vi "LEUI.vi"(0 "LED Update Rate (s)":dbl=0.25 caption="Delay Time (s)", 6 "LEUI_Buttons":T1={"Cycle Selection"=enum."Cycle 0", "SW302 - Option"=TRUE, "SW301 - Start/Pause"=FALSE, "Cycle Selection"=enum."Cycle 0", "Number of positions 1"=2, "Knob Position 1"=0, "Number of positions 2"=2, "Knob Position 2"=0, "Number of positions 3"=2, "Knob Position 3"=0, "Number of positions 4"=2, "Knob Position 4"=0} {"Knob Position 4" items=["Six"=5, "Five"=4, "Four"=3, "Three"=2, "Two"=1, "One"=0]; "Number of positions 4" items=["Six"=5, "Five"=4, "Four"=3, "Three"=2]; "Knob Position 3" items=["Six"=5, "Five"=4, "Four"=3, "Three"=2, "Two"=1, "One"=0]; "Number of positions 3" items=["Six"=5, "Five"=4, "Four"=3, "Three"=2]; "Knob Position 2" items=["Six"=5, "Five"=4, "Four"=3, "Three"=2, "Two"=1, "One"=0]; "Number of positions 2" items=["Six"=5, "Five"=4, "Four"=3, "Three"=2]; "Knob Position 1" items=["Six"=5, "Five"=4, "Four"=3, "Three"=2, "Two"=1, "One"=0]; "Number of positions 1" items=["Six"=5, "Five"=4, "Four"=3, "Three"=2]}, 7 "stop":bool, 11 "Error In":errorcluster) -> (15 "Error Out":errorcluster)   [LabVIEW 2014]
doc: "This VI controls the high end 2015 VA washer UI board. The VI updates the status of the LEDs every 'LED update rate (s)' number of seconds. The VI allows the user to press buttons and select a cycle."
uses:
  Laundry Tool 1.0 Support/type defs/LEUI_Buttons.ctl
  Laundry Tool 1.0 Support/type defs/LEUI_LEDs_SLB.ctl
  Common/LabVIEW GEA2 Toolkit/LabVIEW_GEA2_Toolkit.lvlibp/type defs/Data In.ctl
  Common/LabVIEW GEA2 Toolkit/LabVIEW_GEA2_Toolkit.lvlibp/type defs/Source_Destination.ctl
  Common/LabVIEW GEA2 Toolkit/LabVIEW_GEA2_Toolkit.lvlibp/type defs/ERD Read Data In.ctl
  Common/LabVIEW GEA2 Toolkit/LabVIEW_GEA2_Toolkit.lvlibp/type defs/Data Type.ctl
  Common/LabVIEW GEA2 Toolkit/LabVIEW_GEA2_Toolkit.lvlibp/type defs/ERD Write Data In.ctl
  Automation/Product Specific/Clothes Care/2015 VA Washer/Product Testcode/VALEW/Valew Common/type defs/UI Buttons.ctl
  Automation/Product Specific/Clothes Care/2015 VA Washer/Product Testcode/VALEW/Valew Common/type defs/Encoder Position.ctl
  Common/LabVIEW GEA2 Toolkit/LabVIEW_GEA2_Toolkit.lvlibp
panel:
  in  "Soft Load box?":bool
  out "LEUI_LEDs_Out":T2
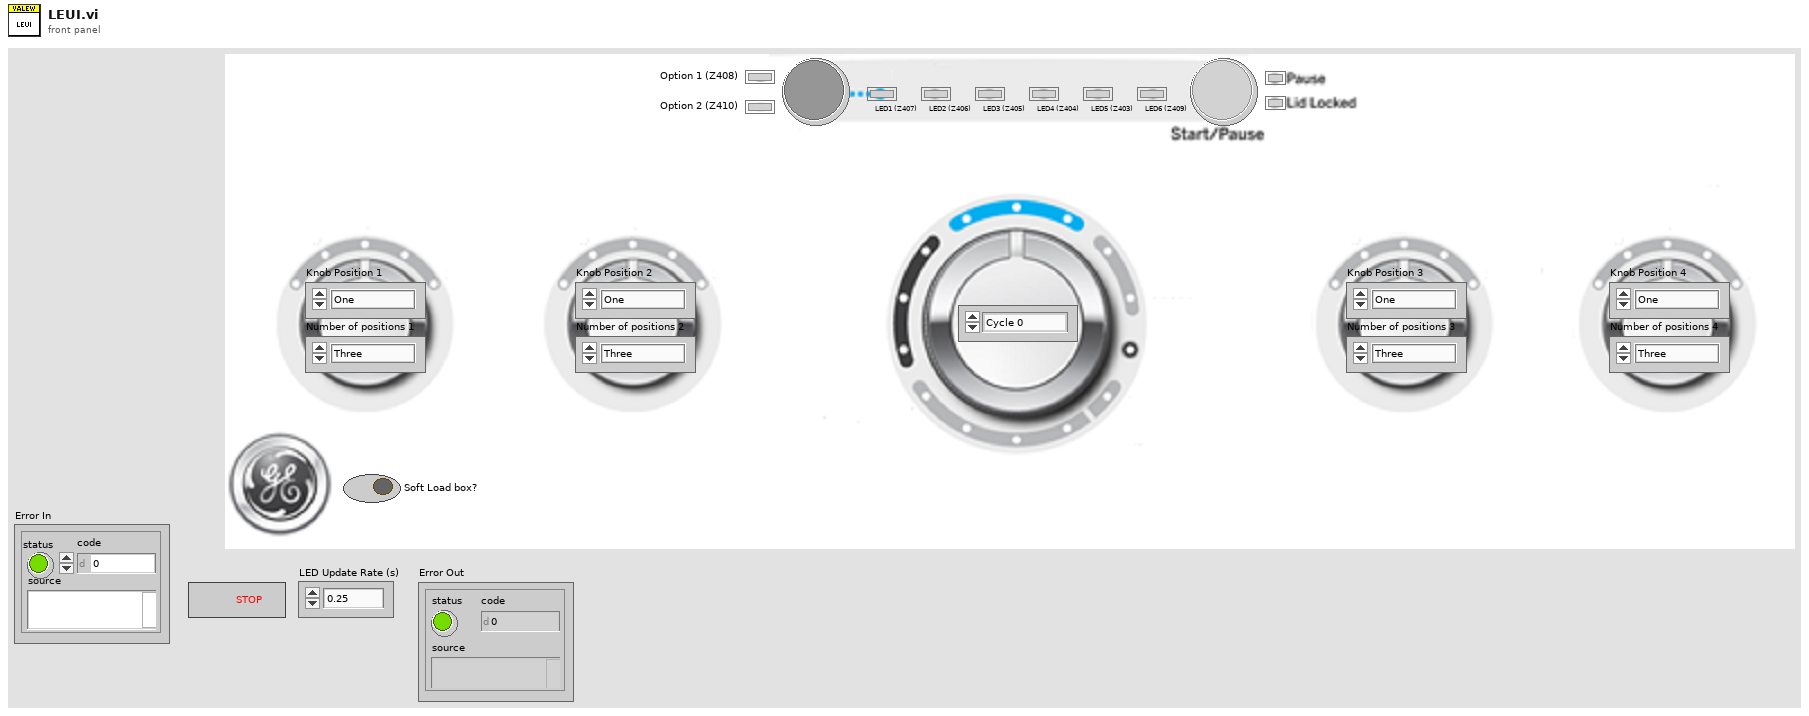
[diagram p1: front panel]
types:
  T1 = typedef "LEUI_Buttons.ctl" = cluster{"Cycle Selection":enum16{"Cycle 0", "Cycle 1", "Cycle 2", "Cycle 3", "Cycle 4", "Cycle 5", "Cycle 6", "Cycle 7", "Cycle 8", "Cycle 9", "Cycle 10", "Cycle 11", "Cycle 12", "Cycle 13"}, "SW302 - Option":bool, "SW301 - Start/Pause":bool, "Cycle Selection":enum16{"Cycle 13", "Cycle 12", "Cycle 11", "Cycle 10", "Cycle 9", "Cycle 8", "Cycle 7", "Cycle 6", "Cycle 5", "Cycle 4", "Cycle 3", "Cycle 2", "Cycle 1", "Cycle 0"}, "Number of positions 1":i32, "Knob Position 1":i32, "Number of positions 2":i32, "Knob Position 2":i32, "Number of positions 3":i32, "Knob Position 3":i32, "Number of positions 4":i32, "Knob Position 4":i32}
  T2 = typedef "LEUI_LEDs_SLB.ctl" = cluster{"Pause (Z401)":bool, "Lid Locked (Z402)":bool, "LED1 (Z407)":bool, "LED2 (Z406)":bool, "LED3 (Z405)":bool, "LED4 (Z404)":bool, "LED5 (Z403)":bool, "LED6 (Z409)":bool, "Option 1 (Z408)":bool, "Option 2 (Z410)":bool}
  T3 = typedef "LabVIEW_GEA2_Toolkit.lvlibp/ERD Write Data In.ctl" = cluster{"ERD Number":u16, "Data Type":T4, "Data":string}
  T4 = typedef "LabVIEW_GEA2_Toolkit.lvlibp/Data Type.ctl" = enum16{"string", "boolean", "uint8_t", "uint16_t", "uint32_t", "uint64_t", "int8_t", "int16_t", "int32_t", "int64_t"}
  T5 = typedef "LabVIEW_GEA2_Toolkit.lvlibp/ERD Read Data In.ctl" = cluster{"ERD Number":u16, "Data Type":T4}
  T6 = typedef "LabVIEW_GEA2_Toolkit.lvlibp/Source_Destination.ctl" = cluster{"Source":u8, "Destination":u8}
  T7 = typedef "LabVIEW_GEA2_Toolkit.lvlibp/Data In.ctl" = cluster{"Source":u8, "Destination":u8, "Command":u8, "Message":string}
  T8 = typedef "UI Buttons.ctl" = enum16{"Switch Off", "SW201 - My Cycle", "SW202 - Delay Wash", "SW203 - Extra Rinse", "SW204 - Signal / Volume", "SW205 - Spin", "SW206 - Deep Rinse / Fab Soft", "SW207 - Soil", "SW208 - Auto Soak", "SW209 - Temp", "SW210 - Warm Rinse", "SW211 - Deep Fill", "SW212 - Stain Remover", "SW213 - Power", "SW222 - Control Lock", "SW214 - Start / Pause", "SW301 - Start/Pause LE", "SW302 - Option Button LE"}
  T9 = typedef "Encoder Position.ctl" = enum16{"Position 0", "Position 1", "Position 2", "Position 3", "Position 4", "Position 5", "Position 6", "Position 7", "Position 8", "Position 9", "Position 10", "Position 11", "Position 12", "Position 13", "Clear / Reset"}
  T10 = enum16{"Cycle 13", "Cycle 12", "Cycle 11", "Cycle 10", "Cycle 9", "Cycle 8", "Cycle 7", "Cycle 6", "Cycle 5", "Cycle 4", "Cycle 3", "Cycle 2", "Cycle 1", "Cycle 0"}
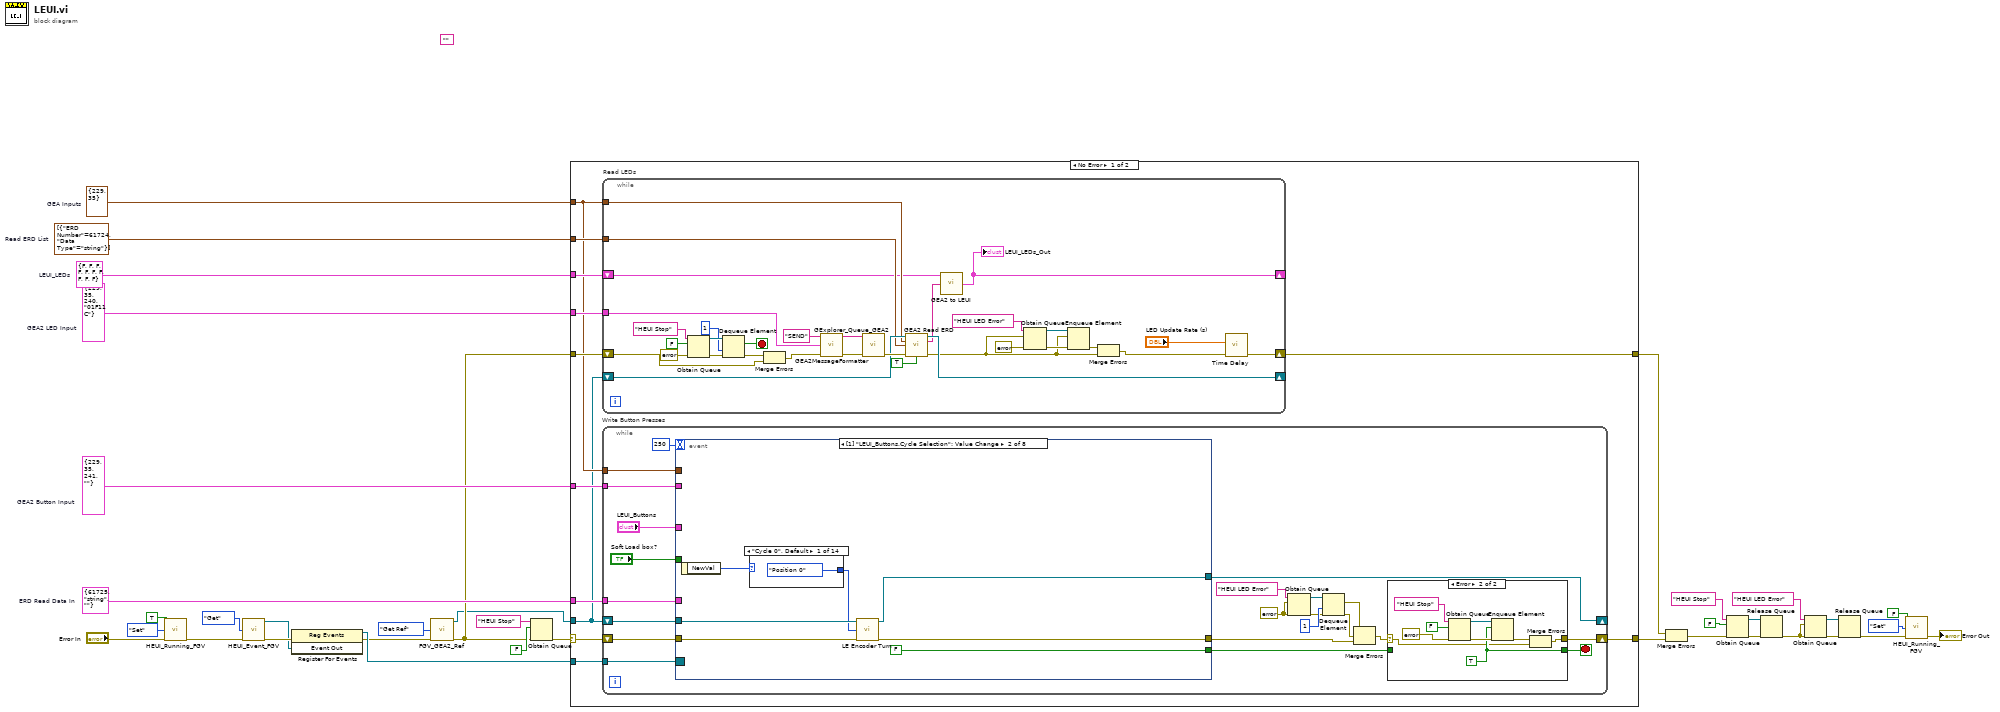
[diagram p0: block diagram]
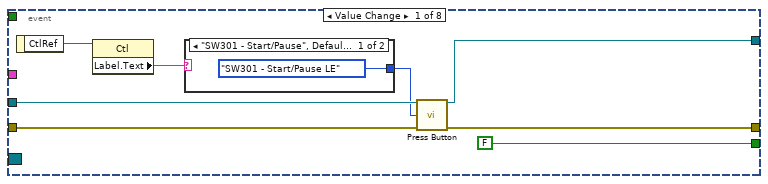
[diagram p3: hidden frame]
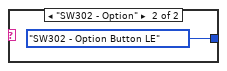
[diagram p4: hidden frame]
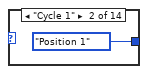
[diagram p5: hidden frame]
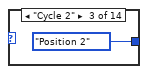
[diagram p6: hidden frame]
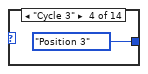
[diagram p7: hidden frame]
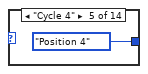
[diagram p8: hidden frame]
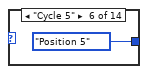
[diagram p9: hidden frame]
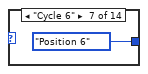
[diagram p10: hidden frame]
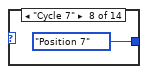
[diagram p11: hidden frame]
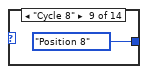
[diagram p12: hidden frame]
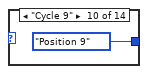
[diagram p13: hidden frame]
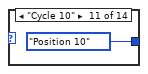
[diagram p14: hidden frame]
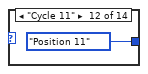
[diagram p15: hidden frame]
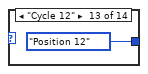
[diagram p16: hidden frame]
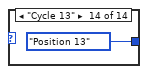
[diagram p17: hidden frame]
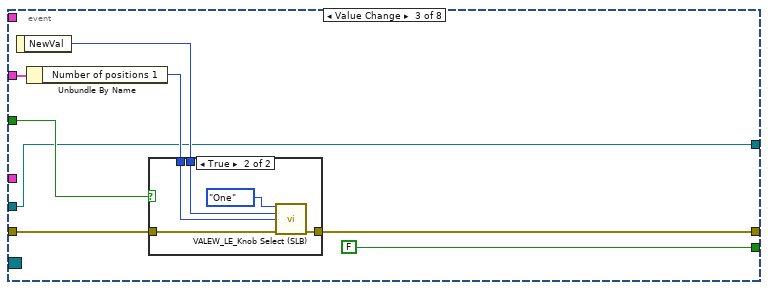
[diagram p18: hidden frame]
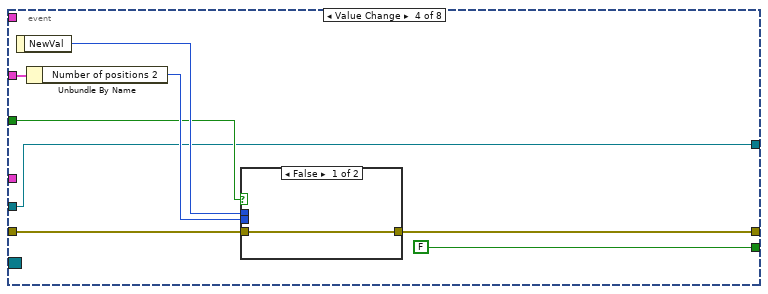
[diagram p20: hidden frame]
diagram:
  w24 = T3 {"ERD Number"=61725, "Data Type"=enum."string", "Data"=""}  # ERD Read Data In
  w26 = T5[] [{"ERD Number"=61724, "Data Type"=enum."string"}]  # Read ERD List
  w25 = T6 {"Source"=229, "Destination"=35}  # GEA Inputs
  w34 = T7 {"Source"=229, "Destination"=35, "Command"=240, "Message"="01F11C"}  # GEA2 LED Input
  w35 = T2 {"Pause (Z401)"=FALSE, "Lid Locked (Z402)"=FALSE, "LED1 (Z407)"=FALSE, "LED2 (Z406)"=FALSE, "LED3 (Z405)"=FALSE, "LED4 (Z404)"=FALSE, "LED5 (Z403)"=FALSE, "LED6 (Z409)"=FALSE, "Option 1 (Z408)"=FALSE, "Option 2 (Z410)"=FALSE}  # LEUI_LEDs
  w33 = T7 {"Source"=229, "Destination"=35, "Command"=241, "Message"=""}  # GEA2 Button Input
  (unwired) ""
  n1 = call "HEUI_Running_FGV.vi"("Running?"=TRUE, "Action"=enum16{"Get", "Set"}."Set", "Error In"="Error In") -> ("Error Out"=w5:errorcluster)  [unwired: 11 in, 1 out]
  n2 = call "HEUI_Event_FGV.vi"("Action"=enum16{"Get", "Set"}."Get", "Error In"=w5) -> ("Event Out"=w15:refnum<user-event>, "Error Out"=w16:errorcluster)  [unwired: 12 in]
  n3 = register-events(error in=w16, w15) -> (reference out=w18:refnum<event-registration>, error out=w11:errorcluster)  [unwired: 1 in]
  n4 = call "FGV_GEA2_Ref.vi"("Action"=enum16{"Set Ref", "Get Ref"}."Get Ref", "Error In"=w11) -> ("GEA2 Reference Out"=w9:refnum<k24>, "Error Out"=w10:errorcluster)  [unwired: 12 in]
  n5 = Obtain Queue(name (unnamed)="HEUI Stop", element data type=FALSE ("stop"), error in (no error)=w10) -> (error out=w23:errorcluster)  [unwired: 2 in, 2 out]
  n6 = case shown="No Error" w23 {
    selector: w23 -> [w38 w225]
    tunnel: w9 -> [w39 _]
    tunnel: [w48 errorcluster {"status"=FALSE, "code"=0, "source"=""} ("error out")] -> w36
    tunnel: [w47 w225] -> w13
    tunnel: w35 -> [w46 _]
    tunnel: w34 -> [w45 _]
    tunnel: w33 -> [w44 _]
    tunnel: w10 -> [w43 _]
    tunnel: w26 -> [w42 _]
    tunnel: w25 -> [w41 _]
    tunnel: w24 -> [w40 _]
    tunnel: w18 -> [w37 _]
    frame No Error {
      n7 = while "Write Button Presses" {
        shift-right: [w96] -> w47
        shift-left: w38 -> [w102]
        shift-right: [w100] -> _
        shift-left: w39 -> [w101]
        tunnel: w44 -> [w99]
        tunnel: w41 -> [w98]
        tunnel: w40 -> [w97]
        tunnel: w37 -> [w83]
        stop <- w94 stop-if-true
        w88 = errorcluster {"status"=FALSE, "code"=0, "source"=""} ("error in (no error)")
        n8 = event shown="[1] \"LEUI_Buttons.Cycle Selection\": Value Change" {
          selector: w83 -> [_ _ _ _ _ _ _ _]
          dyn-events: _ -> [_ _ _ _ _ _ _ _]
          timeout: 250 -> [_ _ _ _ _ _ _ _]
          tunnel: [w114 w124 w148 w162 w176 w190 w219 w222] -> w86
          tunnel: w102 -> [w116 w127 w149 w163 w177 w191 w210 w222]
          tunnel: w101 -> [w118 w128 w145 w160 w174 w188 w201 w223]
          tunnel: [w115 w125 w145 w160 w174 w188 w211 w223] -> w100
          tunnel: [FALSE ("stop") FALSE ("stop") FALSE ("stop") FALSE ("stop") FALSE ("stop") FALSE ("stop") w218 FALSE ("stop")] -> w95
          tunnel: w99 -> [_ _ _ _ _ _ _ _]
          tunnel: w98 -> [_ _ _ _ _ _ w202 _]
          tunnel: w97 -> [_ _ _ _ _ _ _ _]
          tunnel: "LEUI_Buttons" -> [_ _ w152 w166 w180 w194 _ _]
          tunnel: "Soft Load box?" -> [_ _ w146 w161 w175 w189 _ _]
          event Value Change {
            n9 = event-data() -> ("CtlRef"=w121:refnum<vi>)  [unwired: 1 in]
            n10 = property class="Ctl"(reference=w121) -> ("Label.Text"=w119:string)  [unwired: 1 in, 2 out]
            n11 = case shown="\"SW301 - Start/Pause\", Default" w119 {
              tunnel: [UI_Buttons."SW301 - Start/Pause LE" ("Button") UI_Buttons."SW302 - Option Button LE" ("Button")] -> w117
              frame "SW301 - Start/Pause", Default {
              }
              frame "SW302 - Option" {
              }
            }
            n12 = call "Press Button.vi"("GEA2 Reference In"=w118, "Button"=w117, "Error In"=w116) -> ("GEA2 Reference Out"=w115:refnum<k24>, "Error Out"=w114:errorcluster)  [unwired: 11 in]
          }
          event Value Change {
            n13 = event-data() -> ("NewVal"=w129:T10)  [unwired: 1 in]
            n14 = case shown="\"Cycle 0\", Default" w129 {
              tunnel: [Encoder_Position."Position 0" ("Button") Encoder_Position."Position 1" ("Button") Encoder_Position."Position 2" ("Button") Encoder_Position."Position 3" ("Button") Encoder_Position."Position 4" ("Button") Encoder_Position."Position 5" ("Button") Encoder_Position."Position 6" ("Button") Encoder_Position."Position 7" ("Button") Encoder_Position."Position 8" ("Button") Encoder_Position."Position 9" ("Button") Encoder_Position."Position 10" ("Button") Encoder_Position."Position 11" ("Button") Encoder_Position."Position 12" ("Button") Encoder_Position."Position 13" ("Button")] -> w126
              frame "Cycle 0", Default {
              }
              frame "Cycle 1" {
              }
              frame "Cycle 2" {
              }
              frame "Cycle 3" {
              }
              frame "Cycle 4" {
              }
              frame "Cycle 5" {
              }
              frame "Cycle 6" {
              }
              frame "Cycle 7" {
              }
              frame "Cycle 8" {
              }
              frame "Cycle 9" {
              }
              frame "Cycle 10" {
              }
              frame "Cycle 11" {
              }
              frame "Cycle 12" {
              }
              frame "Cycle 13" {
              }
            }
            n15 = call "LE Encoder Turn.vi"("GEA2 Reference In"=w128, "Button"=w126, "Error In"=w127) -> ("GEA2 Reference Out"=w125:refnum<k24>, "Error Out"=w124:errorcluster)  [unwired: 11 in]
          }
          event Value Change {
            n16 = event-data() -> ("NewVal"=w151:i32)  [unwired: 1 in]
            n17 = Unbundle By Name(w152) -> ("Number of positions 1"=w150:i32)
            n18 = case shown="True" w146 {
              tunnel: w151 -> [_ w158]
              tunnel: w150 -> [_ w157]
              tunnel: w149 -> [w153 w155]
              tunnel: [w153 w154] -> w148
              frame False {
              }
              frame True {
                n19 = call "VALEW_LE_Knob Select (SLB).vi"("Knob"=enum16{"One", "Two", "Three", "Four"}."One", "Knob Position"=w158, "Number of positions"=w157, "Error In"=w155) -> ("Error Out"=w154:errorcluster)  [unwired: 11 in]
              }
            }
          }
          event Value Change {
            n20 = event-data() -> ("NewVal"=w165:i32)  [unwired: 1 in]
            n21 = Unbundle By Name(w166) -> ("Number of positions 2"=w164:i32)
            n22 = case shown="False" w161 {
              tunnel: w165 -> [_ w172]
              tunnel: w164 -> [_ w171]
              tunnel: w163 -> [w167 w169]
              tunnel: [w167 w168] -> w162
              frame False {
              }
              frame True {
                n23 = call "VALEW_LE_Knob Select (SLB).vi"("Knob"=enum16{"One", "Two", "Three", "Four"}."Two", "Knob Position"=w172, "Number of positions"=w171, "Error In"=w169) -> ("Error Out"=w168:errorcluster)  [unwired: 11 in]
              }
            }
          }
          event Value Change {
            n24 = event-data() -> ("NewVal"=w179:i32)  [unwired: 1 in]
            n25 = Unbundle By Name(w180) -> ("Number of positions 3"=w178:i32)
            n26 = case shown="True" w175 {
              tunnel: w179 -> [_ w186]
              tunnel: w178 -> [_ w185]
              tunnel: w177 -> [w181 w183]
              tunnel: [w181 w182] -> w176
              frame False {
              }
              frame True {
                n27 = call "VALEW_LE_Knob Select (SLB).vi"("Knob"=enum16{"One", "Two", "Three", "Four"}."Three", "Knob Position"=w186, "Number of positions"=w185, "Error In"=w183) -> ("Error Out"=w182:errorcluster)  [unwired: 11 in]
              }
            }
          }
          event Value Change {
            n28 = event-data() -> ("NewVal"=w193:i32)  [unwired: 1 in]
            n29 = Unbundle By Name(w194) -> ("Number of positions 4"=w192:i32)
            n30 = case shown="True" w189 {
              tunnel: w193 -> [_ w200]
              tunnel: w192 -> [_ w199]
              tunnel: w191 -> [w195 w197]
              tunnel: [w195 w196] -> w190
              frame False {
              }
              frame True {
                n31 = call "VALEW_LE_Knob Select (SLB).vi"("Knob"=enum16{"One", "Two", "Three", "Four"}."Four", "Knob Position"=w200, "Number of positions"=w199, "Error In"=w197) -> ("Error Out"=w196:errorcluster)  [unwired: 11 in]
              }
            }
          }
          event "stop": Value Change; Panel Close; User Event {
            w208 = T3[] [{"ERD Number"=61728, "Data Type"=enum."string", "Data"="0000000000"}] ("Write ERD List")
            w218 = TRUE ("stop")
            n32 = event-data() -> ()  [unwired: 1 in, 1 out]
            n33 = call "Convert Write ERD List to Message.vi"("GEA Inputs"=w202, "Write ERD List"=w208, "Error In"=w210) -> ("GEA Message"=w206:T7, "Error Out"=w207:errorcluster)  [unwired: 11 in]
            n34 = call "GEA2MessageFormatter.vi"("Prefix(Send/Recv)"="SEND", "GEA2 Data In"=w206, "Error In"=w207) -> ("Output String"=w204:string, "Error Out"=w203:errorcluster)  [unwired: 11 in]
            n35 = call "GExplorer_Queue_GEA2.vi"("Output String"=w204, "error in (no error)"=w203) -> ("error out"=w209:errorcluster)  [unwired: 13 in]
            n36 = call "GEA2 Write ERD.vi"("GEA2 Reference In"=w201, "GEA Inputs"=w202, "Write ERD List"=w208, "Error In"=w209) -> ("GEA2 Reference Out"=w211:refnum<k24>, "Error Out"=w212:errorcluster)  [unwired: 9 in, 1 out]
            n37 = control-ref of="This VI"() -> (w220:refnum<vi>)
            n38 = invoke class="VI" method="FP.Close"(reference=w220, error in=w212) -> (error out=w217:errorcluster)  [unwired: 1 in, 2 out]
            n39 = Obtain Queue(name (unnamed)="HEUI Stop", element data type=FALSE ("stop"), error in (no error)=w217) -> (queue out=w215:refnum<queue>, error out=w216:errorcluster)  [unwired: 2 in, 1 out]
            n40 = Enqueue Element(queue=w215, element=w218, error in (no error)=w216) -> (error out=w219:errorcluster)  [unwired: 1 in, 2 out]
          }
          event Timeout {
            n41 = event-data() -> ()  [unwired: 1 in, 3 out]
          }
        }
        n42 = Obtain Queue(name (unnamed)="HEUI LED Error", element data type=w88, error in (no error)=w88) -> (queue out=w90:refnum<queue>, error out=w91:errorcluster)  [unwired: 2 in, 1 out]
        n43 = Dequeue Element(queue=w90, timeout in ms (-1)=1, error in (no error)=w91) -> (element=w84:errorcluster, error out=w85:errorcluster)  [unwired: 2 out]
        n44 = Merge Errors(w84, w85, w86) -> (w89:errorcluster)
        n45 = case shown="Error" w89 {
          selector: w89 -> [w104 w106]
          tunnel: [w104 w108] -> w96
          tunnel: w95 -> [w103 _]
          tunnel: [w103 w109] -> w94
          frame No Error {
          }
          frame Error {
            w109 = TRUE ("stop")
            n46 = Obtain Queue(name (unnamed)="HEUI Stop", element data type=FALSE ("stop"), error in (no error)=errorcluster {"status"=FALSE, "code"=0, "source"=""}) -> (queue out=w112:refnum<queue>, error out=w113:errorcluster)  [unwired: 2 in, 1 out]
            n47 = Enqueue Element(queue=w112, element=w109, error in (no error)=w113) -> (error out=w107:errorcluster)  [unwired: 1 in, 2 out]
            n48 = Merge Errors(w107, w106) -> (w108:errorcluster)
          }
        }
      }
      n49 = while "Read LEDs" {
        shift-right: [w79] -> w48
        shift-left: w43 -> [w50]
        shift-right: [w66] -> _
        shift-left: w39 -> [w65]
        tunnel: w45 -> [w74]
        tunnel: w41 -> [w64]
        tunnel: w42 -> [w63]
        shift-right: [w80] -> _
        shift-left: w46 -> [w49]
        stop <- w73 stop-if-true
        n50 = Obtain Queue(name (unnamed)="HEUI Stop", element data type=FALSE ("stop"), error in (no error)=errorcluster {"status"=FALSE, "code"=0, "source"=""}) -> (queue out=w72:refnum<queue>, error out=w71:errorcluster)  [unwired: 2 in, 1 out]
        n51 = Dequeue Element(queue=w72, timeout in ms (-1)=1, error in (no error)=w71) -> (element=w73:bool, error out=w53:errorcluster)  [unwired: 2 out]
        n52 = Merge Errors(w53, w50) -> (w52:errorcluster)
        n53 = call "GEA2MessageFormatter.vi"("Prefix(Send/Recv)"="SEND", "GEA2 Data In"=w74, "Error In"=w52) -> ("Output String"=w76:string, "Error Out"=w75:errorcluster)  [unwired: 11 in]
        n54 = call "GExplorer_Queue_GEA2.vi"("Output String"=w76, "error in (no error)"=w75) -> ("error out"=w67:errorcluster)  [unwired: 13 in]
        n55 = call "GEA2 Read ERD.vi"("GEA2 Reference In"=w65, "GEA Inputs"=w64, "Read ERD List"=w63, "Error In"=w67, "Verify ERD Response?"=TRUE) -> ("GEA2 Reference Out"=w66:refnum<k24>, "Raw Data Out"=w62:string, "Error Out"=w56:errorcluster)  [unwired: 7 in, 1 out]
        n56 = call "GEA2 to LEUI.vi"("LEUI_LEDs_In"=w49, "Raw Data In"=w62) -> ("LEUI_LEDs_Out"=w80:T2)  [unwired: 13 in]
        "LEUI_LEDs_Out" <- w80
        n57 = Obtain Queue(name (unnamed)="HEUI LED Error", element data type=w56, error in (no error)=errorcluster {"status"=FALSE, "code"=0, "source"=""}) -> (queue out=w59:refnum<queue>, error out=w58:errorcluster)  [unwired: 2 in, 1 out]
        n58 = Enqueue Element(queue=w59, element=w56, error in (no error)=w58) -> (error out=w57:errorcluster)  [unwired: 1 in, 2 out]
        n59 = Merge Errors(w57, w56) -> (w55:errorcluster)
        n60 = call "Time Delay"("error in (no error)"=w55, "Delay Time (s)"="LED Update Rate (s)") -> ("error out"=w79:errorcluster)  [unwired: 9 in]
      }
    }
    frame Error {
    }
  }
  n61 = Merge Errors(w36, w13) -> (w14:errorcluster)
  n62 = Obtain Queue(name (unnamed)="HEUI Stop", element data type=FALSE ("stop"), error in (no error)=w14) -> (queue out=w27:refnum<queue>, error out=w28:errorcluster)  [unwired: 2 in, 1 out]
  n63 = Release Queue(queue=w27, error in (no error)=w28) -> (error out=w19:errorcluster)  [unwired: 1 in, 2 out]
  n64 = Obtain Queue(name (unnamed)="HEUI LED Error", element data type=w19, error in (no error)=w19) -> (queue out=w22:refnum<queue>, error out=w21:errorcluster)  [unwired: 2 in, 1 out]
  n65 = Release Queue(queue=w22, error in (no error)=w21) -> (error out=w2:errorcluster)  [unwired: 1 in, 2 out]
  n66 = call "HEUI_Running_FGV.vi"("Running?"=FALSE, "Action"=enum16{"Get", "Set"}."Set", "Error In"=w2) -> ("Error Out"=→"Error Out":errorcluster)  [unwired: 11 in, 1 out]
